vi "Internal Transition.vi"(8 "error in (no error)":errorcluster, 10 "Context in":refnum<class "Context.lvclass">, 11 "State in":refnum<class "State.lvclass">) -> (0 "error out":errorcluster, 2 "Context out":refnum<class "Context.lvclass">, 3 "State out":refnum<class "State.lvclass">)   [LabVIEW 2024, in "State.lvlib" / "State.lvclass"]
uses:
  State.lvclass
  State.lvclass/State.ctl
  Context/Context/Context.lvclass
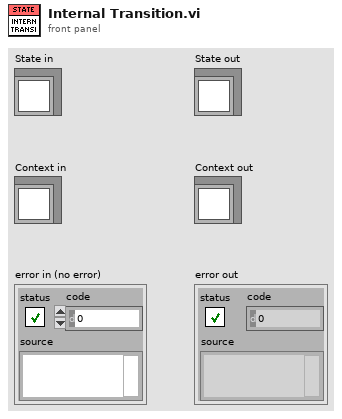
[diagram p1: front panel]
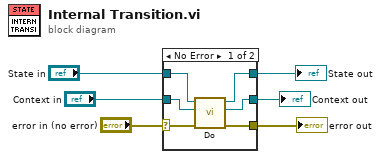
[diagram p0: block diagram]
diagram:
  n1 = case shown="No Error" "error in (no error)" {
    selector: "error in (no error)" -> [w9 w15]
    tunnel: [w8 w15] -> w5
    tunnel: [w10 w14] -> w3
    tunnel: "State in" -> [w12 w14]
    tunnel: [w11 w13] -> w1
    tunnel: "Context in" -> [w7 w13]
    frame No Error {
      n2 = call-dynamic "Do.vi"("error in (no error)"=w9, "Context in"=w7, "State in"=w12) -> ("error out"=w8:errorcluster, "Context out"=w11:refnum<class "Context.lvclass">, "State out"=w10:refnum<class "State.lvclass">)  [unwired: 6 in]
    }
    frame Error {
    }
  }
  "error out" <- w5
  "State out" <- w3
  "Context out" <- w1
